vi "BuildWave-DPO4000.vi"(12 "Input Parameters":T2 {"Data Width" items=["1", "2"]; "Channel" items=["Channel 1", "Channel 2", "Channel 3", "Channel 4", "Math", "Reference 1", "Reference 2", "Reference 3", "Reference 4"]}) -> (1 "Waveform \nConstruction":T1)   [LabVIEW 2014]
doc: "Program queries data from the Tektronix DPO 4000 series oscilloscope and assembles the waveform."
panel:
  out "PT_Off":ext format="%.2e"
  out "Xzero":ext format="%.2e"
  out "Yzero":ext format="%.2e"
  out "Xincr":ext format="%.2e"
  out "Ymult":ext format="%.2e"
  out "Yoff":ext format="%.2e"
  out "Waveform Array":dbl[](array[numeric])
  # "This program reads binary data from a Tektronix DPO4000 series oscilloscope to construct waveform values for a 10 MeV LINAC pulse."
  # "SCOPE VARIABLES"
  # "WAVEFORM CONSTRUCTION"
  # "INPUT PARAMETERS"
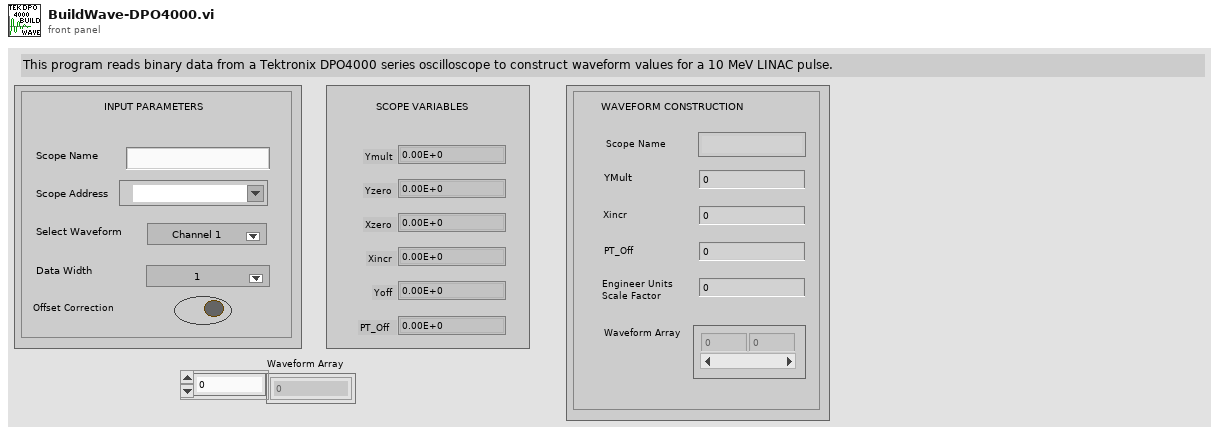
[diagram p1: front panel]
types:
  T1 = cluster{"Scope Name":string, "YMult":dbl, "Xincr":dbl, "PT_Off":dbl, "Engineer Units\nScale Factor":dbl, "Waveform Array":dbl[]}
  T2 = cluster{"Scope Address":refnum<visa-resource-name>, "Channel":u8, "Data Width":u8, "Offset Correction":bool, "Scope Name":string}
  T3 = cluster{"Scope Name":string, dbl, dbl, dbl, "Engineering Format Scale Factor":dbl, dbl[]}
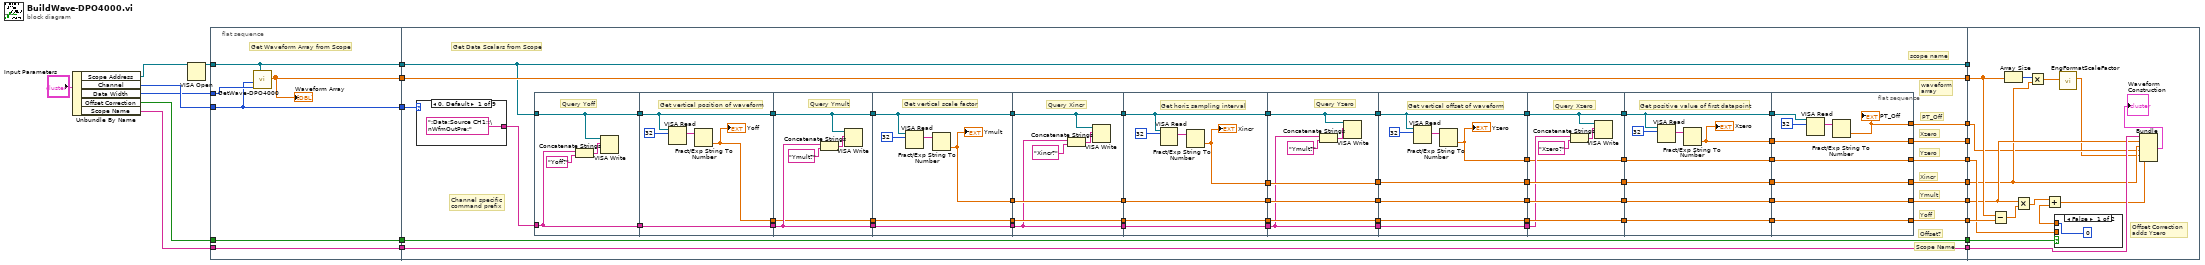
[diagram p0: block diagram]
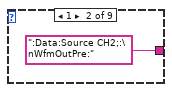
[diagram p2: hidden frame]
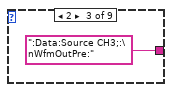
[diagram p3: hidden frame]
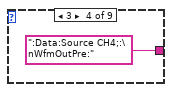
[diagram p4: hidden frame]
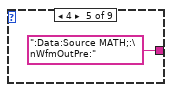
[diagram p5: hidden frame]
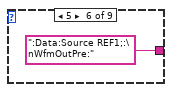
[diagram p6: hidden frame]
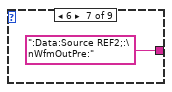
[diagram p7: hidden frame]
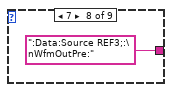
[diagram p8: hidden frame]
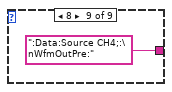
[diagram p9: hidden frame]
diagram:
  n1 = Unbundle By Name("Input Parameters") -> ("Scope Address"=w9:refnum<visa-resource-name>, "Channel"=w8:u8, "Data Width"=w7:u8, "Offset Correction"=w6:bool, "Scope Name"=w5:string)
  n2 = VISA Open(VISA resource name=w9) -> (VISA resource name=w22:refnum<visa-resource-name>)  [unwired: 4 in, 1 out]
  n3 = flat-sequence {
    tunnel: w22 -> [w27]
    tunnel: w7 -> [w28]
    tunnel: w8 -> [w25]
    tunnel: [w27] -> w21
    tunnel: [w26] -> w20
    tunnel: [w25] -> w19
    tunnel: w6 -> [w23]
    tunnel: w5 -> [w24]
    tunnel: [w24] -> w4
    tunnel: [w23] -> w3
    tunnel: w21 -> [w79]
    tunnel: w20 -> [w82]
    tunnel: w19 -> [w83]
    tunnel: [w82] -> w18
    tunnel: [w79] -> w17
    tunnel: [w42] -> w16
    tunnel: [w41] -> w15
    tunnel: [w40] -> w14
    tunnel: [w39] -> w13
    tunnel: [w38] -> w12
    tunnel: [w31] -> w11
    tunnel: w4 -> [w29]
    tunnel: w3 -> [w30]
    tunnel: [w30] -> w2
    tunnel: [w29] -> w1
    tunnel: w18 -> [w179]
    tunnel: w17 -> [_]
    tunnel: w16 -> [_]
    tunnel: w15 -> [w174]
    tunnel: w14 -> [w170]
    tunnel: w13 -> [w171]
    tunnel: w12 -> [w178]
    tunnel: w11 -> [w169]
    tunnel: w2 -> [w176]
    tunnel: w1 -> [w172]
    frame #0 {
      # "Get Waveform Array from Scope"
      n4 = call "GetWave-DPO4000.vi"("Channel"=w25, "Data Width"=w28, "Scope"=w27) -> ("Waveform Array"=w26:dbl[])  [unwired: 7 in]
      "Waveform Array" <- w26
    }
    frame #1 {
      # "Scope Name"
      # "Offset?"
      # "PT_Off"
      # "scope name"
      # "waveform\narray"
      # "Xzero"
      # "Yzero"
      # "Xincr"
      # "Ymult"
      # "Yoff"
      # "Channel specific \ncommand prefix"
      # "Get Data Scalars from Scope"
      n5 = case shown="0, Default" w83 {
        tunnel: [":Data:Source CH1;:\nWfmOutPre:" ":Data:Source CH2;:\nWfmOutPre:" ":Data:Source CH3;:\nWfmOutPre:" ":Data:Source CH4;:\nWfmOutPre:" ":Data:Source MATH;:\nWfmOutPre:" ":Data:Source REF1;:\nWfmOutPre:" ":Data:Source REF2;:\nWfmOutPre:" ":Data:Source REF3;:\nWfmOutPre:" ":Data:Source CH4;:\nWfmOutPre:"] -> w81
        frame 0, Default {
        }
        frame 1 {
        }
        frame 2 {
        }
        frame 3 {
        }
        frame 4 {
        }
        frame 5 {
        }
        frame 6 {
        }
        frame 7 {
        }
        frame 8 {
        }
      }
      n6 = flat-sequence {
        tunnel: w81 -> [w87]
        tunnel: [w87] -> w80
        tunnel: w79 -> [w84]
        tunnel: [w84] -> w78
        tunnel: w80 -> [w92]
        tunnel: w78 -> [w91]
        tunnel: [w91] -> w74
        tunnel: [w92] -> w70
        tunnel: [w88] -> w69
        tunnel: [w94] -> w75
        tunnel: w74 -> [w94]
        tunnel: [w97] -> w71
        tunnel: w70 -> [w97]
        tunnel: w69 -> [w93]
        tunnel: [w93] -> w65
        tunnel: [w101] -> w76
        tunnel: w75 -> [w101]
        tunnel: [w103] -> w72
        tunnel: w71 -> [w103]
        tunnel: [w99] -> w68
        tunnel: [w98] -> w66
        tunnel: w65 -> [w98]
        tunnel: [w104] -> w77
        tunnel: w76 -> [w104]
        tunnel: [w107] -> w73
        tunnel: w72 -> [w107]
        tunnel: w68 -> [w108]
        tunnel: [w109] -> w67
        tunnel: w66 -> [w109]
        tunnel: [w108] -> w64
        tunnel: [w111] -> w63
        tunnel: w77 -> [w111]
        tunnel: [w116] -> w61
        tunnel: w73 -> [w116]
        tunnel: [w115] -> w59
        tunnel: w67 -> [w115]
        tunnel: [w114] -> w57
        tunnel: w64 -> [w114]
        tunnel: [w110] -> w54
        tunnel: w63 -> [w117]
        tunnel: [w117] -> w62
        tunnel: w61 -> [w120]
        tunnel: [w120] -> w60
        tunnel: w59 -> [w123]
        tunnel: [w123] -> w58
        tunnel: w57 -> [w122]
        tunnel: [w122] -> w56
        tunnel: [w121] -> w55
        tunnel: w54 -> [w121]
        tunnel: w62 -> [w124]
        tunnel: [w124] -> w53
        tunnel: w60 -> [w131]
        tunnel: [w131] -> w51
        tunnel: w58 -> [w130]
        tunnel: [w130] -> w50
        tunnel: w56 -> [w129]
        tunnel: [w129] -> w48
        tunnel: [w128] -> w46
        tunnel: w55 -> [w128]
        tunnel: [w127] -> w44
        tunnel: w53 -> [w133]
        tunnel: [w133] -> w52
        tunnel: w51 -> [w135]
        tunnel: w50 -> [w139]
        tunnel: [w139] -> w49
        tunnel: w48 -> [w138]
        tunnel: [w138] -> w47
        tunnel: w46 -> [w137]
        tunnel: [w137] -> w45
        tunnel: w44 -> [w132]
        tunnel: [w132] -> w43
        tunnel: w52 -> [w140]
        tunnel: w49 -> [w143]
        tunnel: w47 -> [w144]
        tunnel: w45 -> [w145]
        tunnel: w43 -> [w142]
        tunnel: [w145] -> w37
        tunnel: [w144] -> w36
        tunnel: [w143] -> w35
        tunnel: [w142] -> w34
        tunnel: [w141] -> w33
        tunnel: [w140] -> w32
        tunnel: [w152] -> w42
        tunnel: [w153] -> w41
        tunnel: [w154] -> w38
        tunnel: [w155] -> w39
        tunnel: [w156] -> w40
        tunnel: w37 -> [w156]
        tunnel: w36 -> [w155]
        tunnel: w35 -> [w154]
        tunnel: w34 -> [w153]
        tunnel: w33 -> [w152]
        tunnel: w32 -> [w149]
        tunnel: [w148] -> w31
        frame #0 {
          # "Query Yoff"
          n7 = Concatenate Strings(w87, "Yoff?") -> (w85:string)
          n8 = VISA Write(VISA resource name=w84, write buffer=w85) -> ()  [unwired: 1 in, 3 out]
        }
        frame #1 {
          # "Get vertical position of waveform"
          n9 = VISA Read(VISA resource name=w91, byte count=32) -> (read buffer=w89:string)  [unwired: 1 in, 3 out]
          n10 = Fract/Exp String To Number(string=w89) -> (number=w88:dbl)  [unwired: 3 in, 1 out]
          "Yoff" <- w88
        }
        frame #2 {
          # "Query Ymult"
          n11 = Concatenate Strings(w97, "Ymult?") -> (w95:string)
          n12 = VISA Write(VISA resource name=w94, write buffer=w95) -> ()  [unwired: 1 in, 3 out]
        }
        frame #3 {
          # "Get vertical scale factor"
          n13 = VISA Read(VISA resource name=w101, byte count=32) -> (read buffer=w100:string)  [unwired: 1 in, 3 out]
          n14 = Fract/Exp String To Number(string=w100) -> (number=w99:dbl)  [unwired: 3 in, 1 out]
          "Ymult" <- w99
        }
        frame #4 {
          # "Query Xincr"
          n15 = Concatenate Strings(w107, "Xincr?") -> (w105:string)
          n16 = VISA Write(VISA resource name=w104, write buffer=w105) -> ()  [unwired: 1 in, 3 out]
        }
        frame #5 {
          # "Get horiz sampling interval"
          n17 = VISA Read(VISA resource name=w111, byte count=32) -> (read buffer=w112:string)  [unwired: 1 in, 3 out]
          n18 = Fract/Exp String To Number(string=w112) -> (number=w110:dbl)  [unwired: 3 in, 1 out]
          "Xincr" <- w110
        }
        frame #6 {
          # "Query Yzero"
          n19 = Concatenate Strings(w120, "Ymult?") -> (w118:string)
          n20 = VISA Write(VISA resource name=w117, write buffer=w118) -> ()  [unwired: 1 in, 3 out]
        }
        frame #7 {
          # "Get vertical offset of waveform"
          n21 = VISA Read(VISA resource name=w124, byte count=32) -> (read buffer=w126:string)  [unwired: 1 in, 3 out]
          n22 = Fract/Exp String To Number(string=w126) -> (number=w127:dbl)  [unwired: 3 in, 1 out]
          "Yzero" <- w127
        }
        frame #8 {
          # "Query Xzero"
          n23 = Concatenate Strings(w135, "Xzero?") -> (w134:string)
          n24 = VISA Write(VISA resource name=w133, write buffer=w134) -> ()  [unwired: 1 in, 3 out]
        }
        frame #9 {
          # "Get positive value of first datapoint"
          n25 = VISA Read(VISA resource name=w140, byte count=32) -> (read buffer=w146:string)  [unwired: 1 in, 3 out]
          n26 = Fract/Exp String To Number(string=w146) -> (number=w141:dbl)  [unwired: 3 in, 1 out]
          "Xzero" <- w141
        }
        frame #10 {
          n27 = VISA Read(VISA resource name=w149, byte count=32) -> (read buffer=w150:string)  [unwired: 1 in, 3 out]
          n28 = Fract/Exp String To Number(string=w150) -> (number=w148:dbl)  [unwired: 3 in, 1 out]
          "PT_Off" <- w148
        }
      }
    }
    frame #2 {
      # "Offset Correction\nadds Yzero"
      n29 = Subtract(x=w179, y=w178) -> (x-y=w177:dbl[])
      n30 = Array Size(array=w179) -> (size(s)=w181:i32)
      n31 = Multiply(x=w171, y=w177) -> (x*y=w175:dbl[])
      n32 = Multiply(x=w181, y=w170) -> (x*y=w180:dbl)
      n33 = case shown="False" w176 {
        tunnel: w174 -> [_ w183]
        tunnel: [0 w183] -> w173
        frame False {
        }
        frame True {
        }
      }
      n34 = Add(x=w175, y=w173) -> (x+y=w167:dbl[])
      n35 = call "EngFormatScaleFactor.vi"("Input Number"=w180) -> ("Engineering Format Scale Factor"=w168:dbl)  [unwired: 10 in]
      n36 = Bundle("Scope Name"=w172, w171, w170, w169, "Engineering Format Scale Factor"=w168, w167) -> (→"Waveform \nConstruction":T3)  [unwired: 1 in]
    }
  }
